vi "2022NewInstrumentationU6_SINGLE_CHANNEL_TEST.vi"() -> ()   [LabVIEW 2021]
panel:
  out "Test 2":dbl(graph)
  in  "Binary 2":bool
  in  "AIN Range":u16(ring) items=["LJ_rgBIP10V", "LJ_rgBIP1V", "LJ_rgBIPP1V", "LJ_rgBIPP01V"]
  in  "FirstFound":bool=TRUE
  in  "Address":string="1"
  out "Error Message 2":string="No Error"
  out "error out":errorcluster
  out "Cold Junction Temp":dbl=41420.0 format="%.6f"
  out "Test":dbl(graph)
  in  "Iterations/Second":i32=1
  in  "Binary":bool
  in  "StreamSettlingFactor":i32
  in  "Resolution Index":u8
  in  "Range Constants":u8[](array[ring])=[0, 0, 0, 0] items=["LJ_rgBIP10V", "LJ_rgBIP1V", "LJ_rgBIPP1V", "LJ_rgBIPP01V"]
  out "Stream Parameters":T1 {"Device Backlog [%]" format="%.2f"}
  in  "PC buffer size (seconds)":dbl=10.0 format="%.2f"
  out "# of iterations":i32
  in  "Scan Rate (Hz)":dbl=1000.0 format="%.3f"
  in  "stop":bool
  out "Error Message":string
  # "This example streams from the first found USB U6."
  # "Data Output For Pressure, Temperature, and Load Sensors"
  # "The + scan list is the positive\nchannels.  For each element in\nthe + list, there must also be\nan element in the - list, which is\nthe negative channels.  For\nsingle-ended channels, put in\n199 for the negative channel.\n\nTo remove an element, right-click\non it, select Data Operations =>\nRemove Element.\n\nTo empty an array, right-click\nnear the edge, select Data\nOperations => Empty Array.\n\nOther useful operations:  From the\nOperate menu are \"Make Current\nValues Default\" and \"Reinitialize\nTo Default\"."
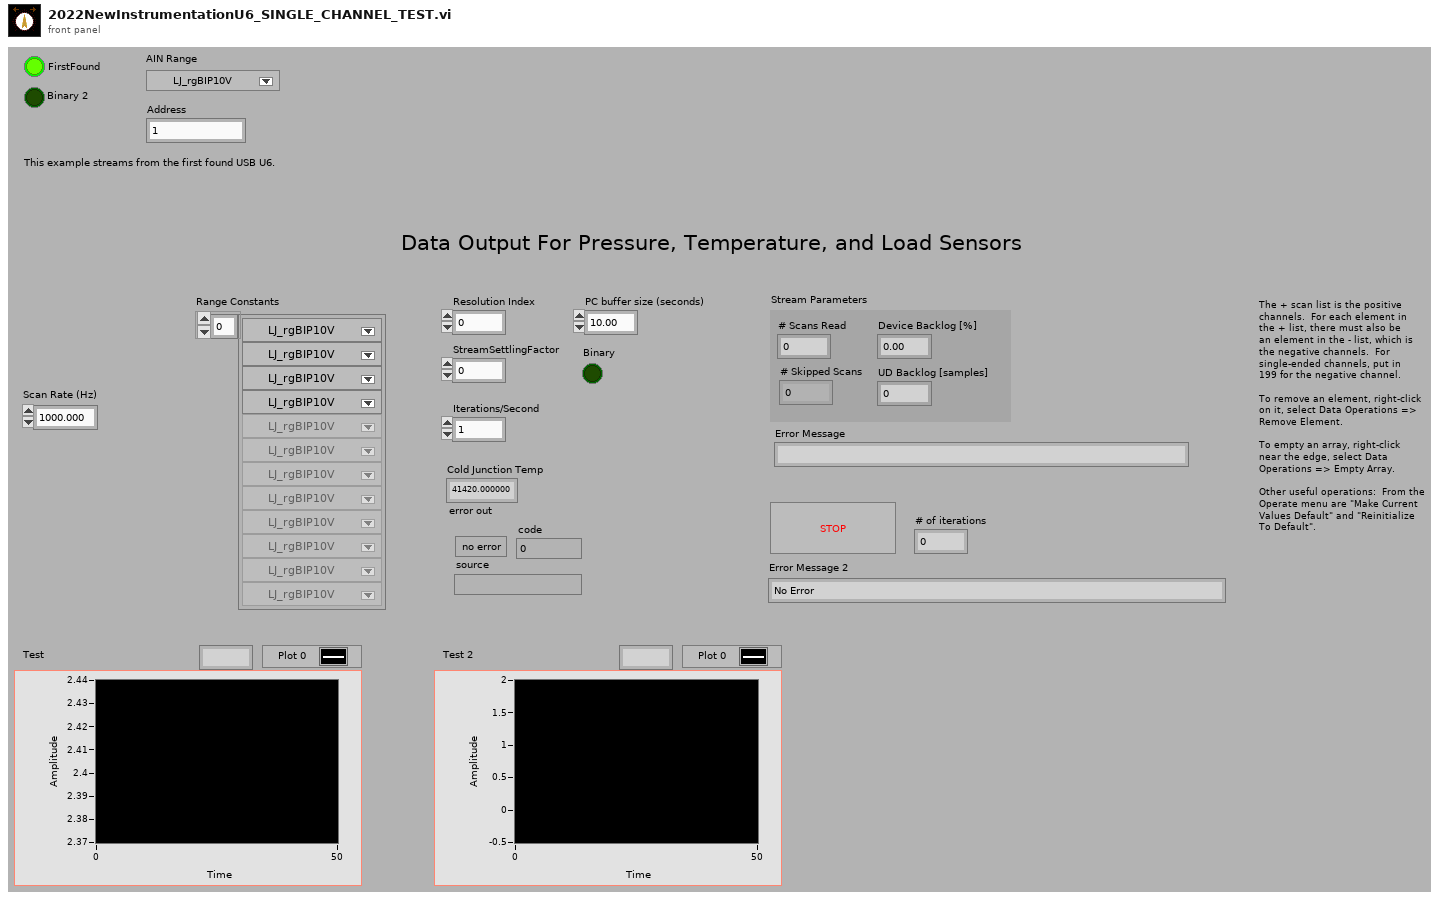
[diagram p1: front panel]
types:
  T1 = cluster{"# Scans Read":i32, "# Skipped Scans":i32, "Device Backlog [%]":dbl, "UD Backlog [samples]":i32}
  T2 = cluster{"PC buffer size (seconds)":dbl, "Resolution Index":u8, "StreamSettlingFactor":i32, "Binary":bool}
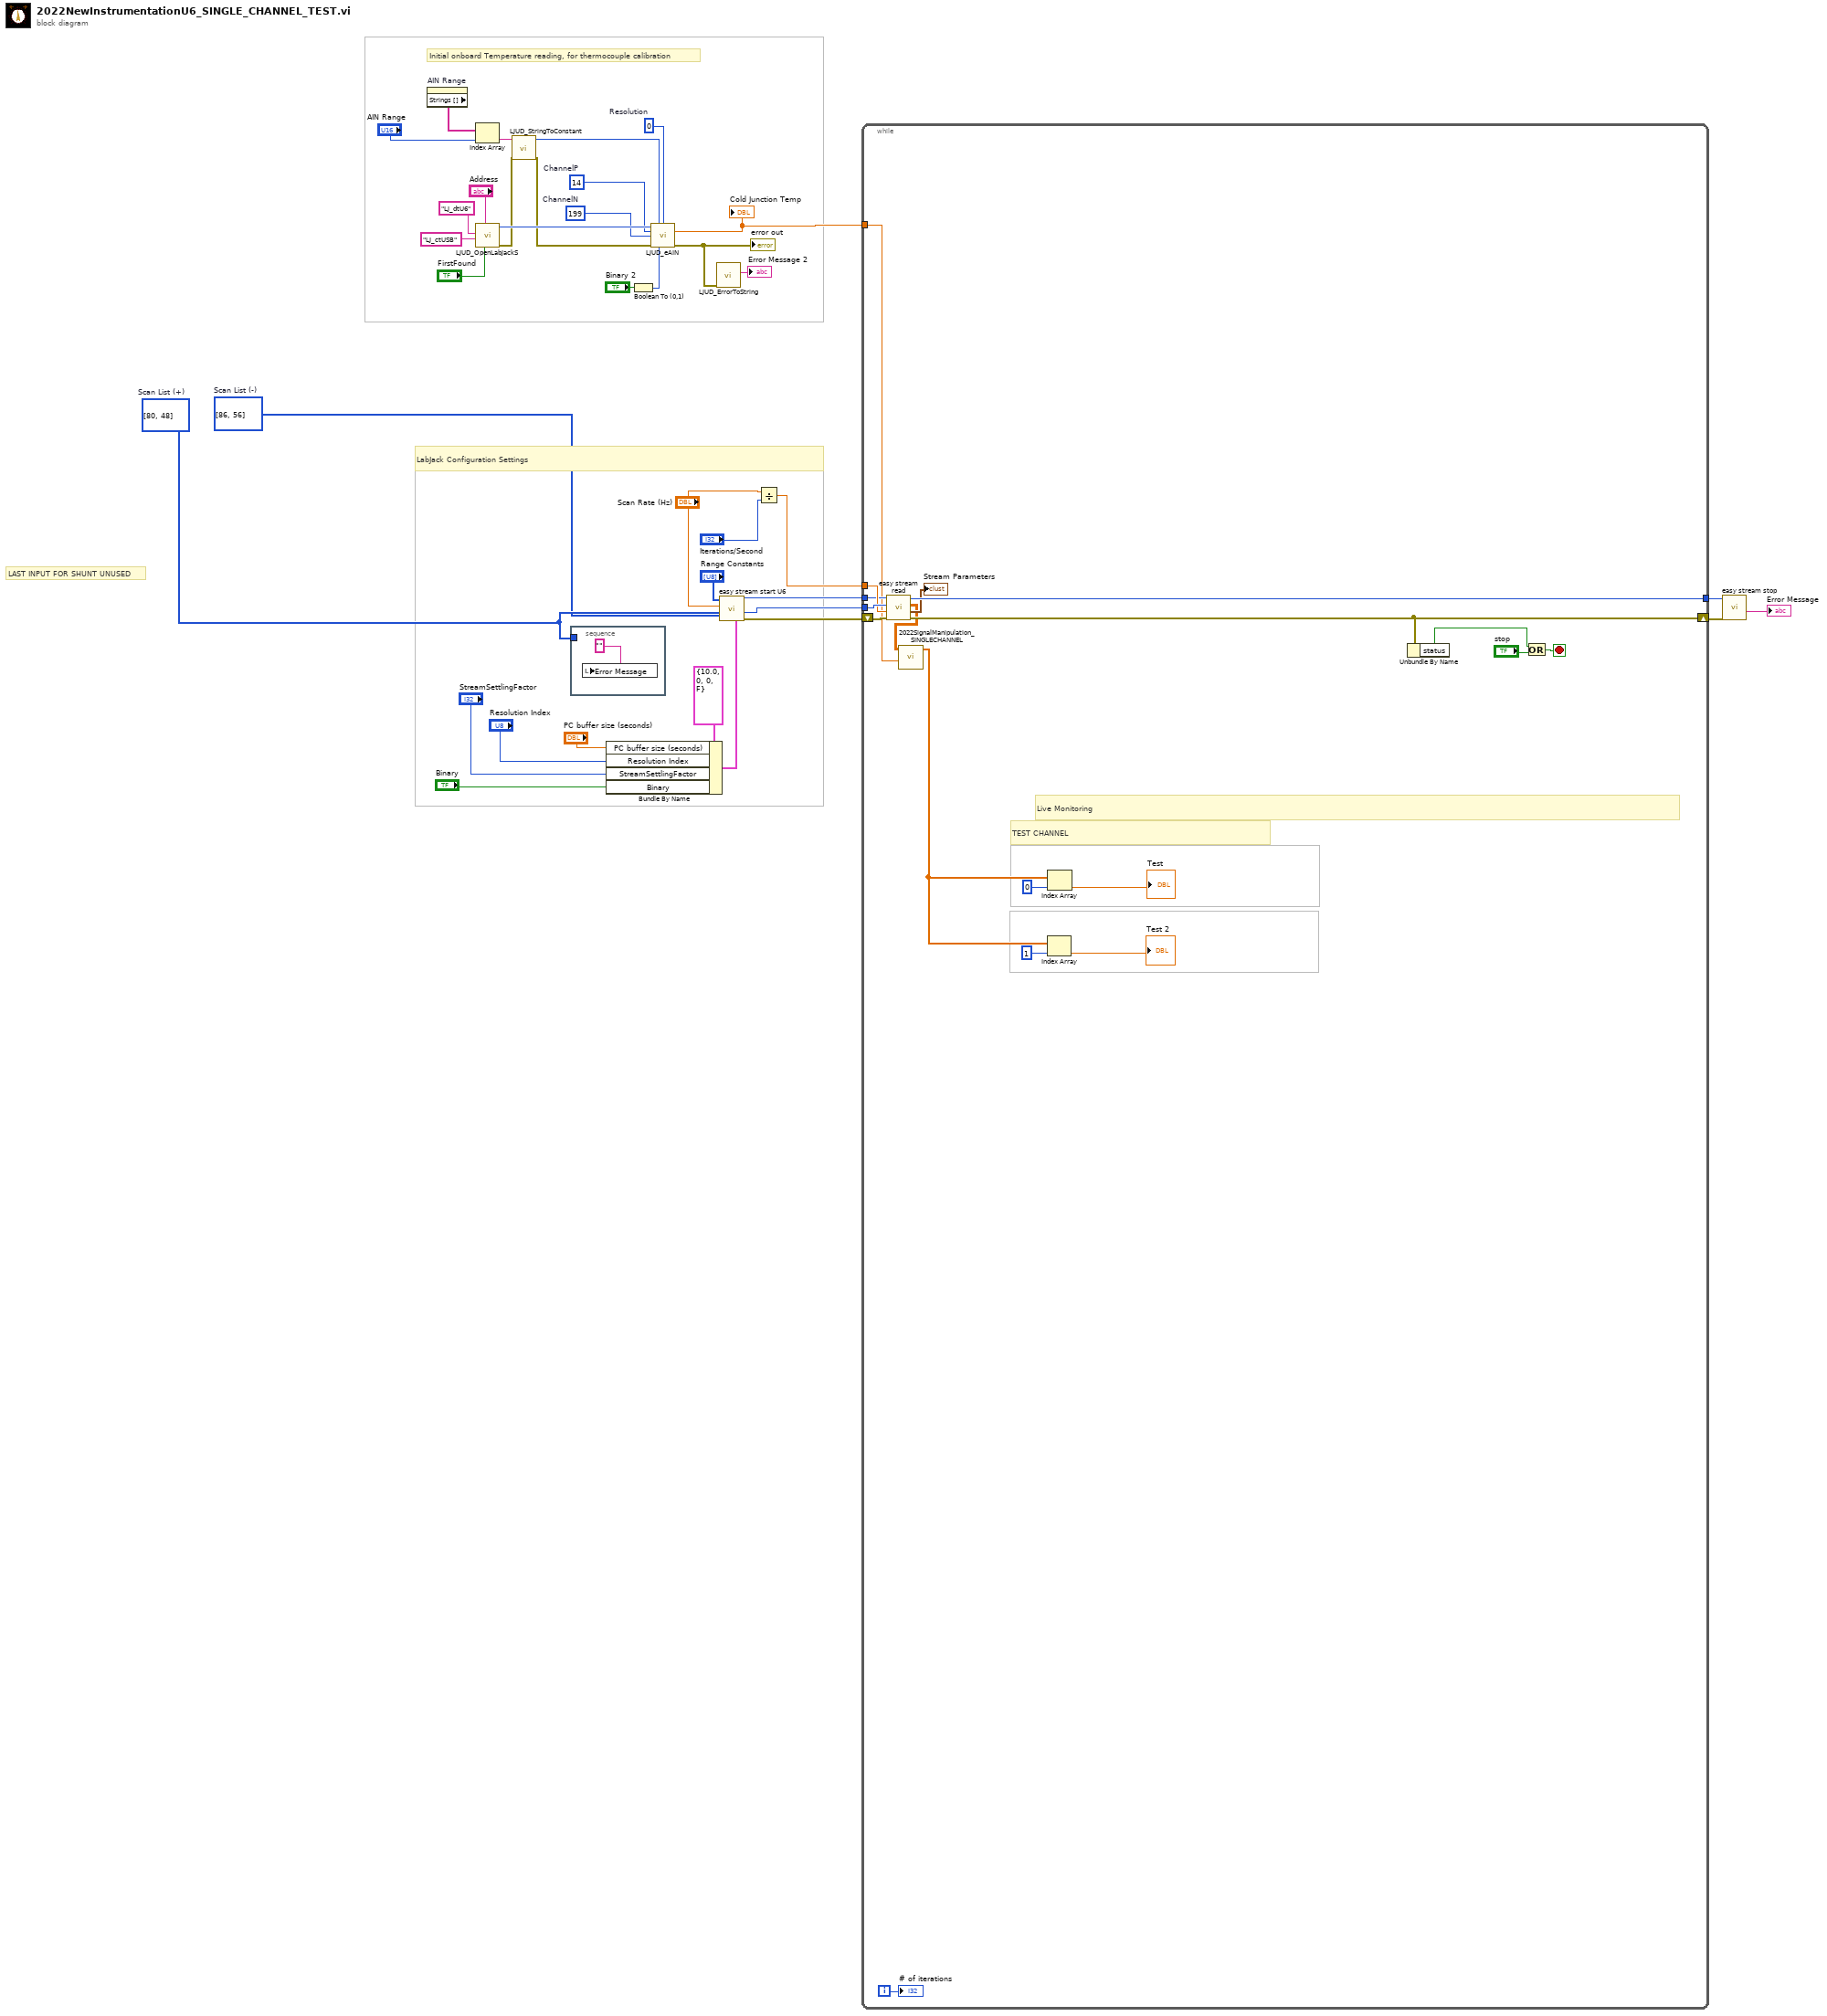
[diagram p0: block diagram]
diagram:
  w12 = 0  # Resolution
  w2 = 199  # ChannelN
  w3 = 14  # ChannelP
  w20 = i32[] [86, 56]  # Scan List (-)
  w21 = i32[] [80, 48]  # Scan List (+)
  # "LAST INPUT FOR SHUNT UNUSED"
  # "LabJack Configuration Settings"
  # "Initial onboard Temperature reading, for thermocouple calibration"
  n1 = property on="AIN Range" class="Ring (strict)"() -> ("Strings []"=w8:string[])  [unwired: 2 in, 2 out]
  n2 = Index Array(array=w8, index="AIN Range") -> (element=w6:string)
  n3 = call "LJUD_OpenLabJackS.vi"("FirstFound"="FirstFound", "Address"="Address", "ConnectionType"="LJ_ctUSB", "DeviceType"="LJ_dtU6") -> ("error out"=w11:errorcluster, "Handle"=w15:i32)  [unwired: 5 in, 1 out]
  n4 = call "LJUD_StringToConstant.vi"("error in"=w11, "String"=w6) -> ("error out"=w10:errorcluster, "Constant Number"=w13:i32)  [unwired: 8 in]
  n5 = stacked-sequence {
    tunnel: w21 -> [_]
    frame #0 {
      n6 = local write "Error Message"("" ("Error Message")) -> ()
    }
  }
  n7 = Bundle By Name(cluster=T2 {"PC buffer size (seconds)"=10.0, "Resolution Index"=0, "StreamSettlingFactor"=0, "Binary"=FALSE} ("Advanced"), "PC buffer size (seconds)"="PC buffer size (seconds)", "Resolution Index"="Resolution Index", "StreamSettlingFactor"="StreamSettlingFactor", "Binary"="Binary") -> (w28:T2)
  n8 = Boolean To (0,1)(Boolean="Binary 2") -> (0, 1=w4:i16)
  n9 = call "LJUD_eAIN.vi"("Handle In"=w15, "Range"=w13, "Resolution"=w12, "ChannelP"=w3, "ChannelN"=w2, "error in"=w10, "Binary"=w4) -> ("Voltage"=w1:dbl, "error out"=w18:errorcluster)  [unwired: 6 in, 1 out]
  "Cold Junction Temp" <- w1
  "error out" <- w18
  n10 = call "LJUD_ErrorToString.vi"("error in"=w18) -> ("String"=→"Error Message 2":string)  [unwired: 10 in]
  n11 = call "easy stream start U6.vi"("Advanced"=w28, "Scan List (-)"=w20, "Scan List (+)"=w21, "Scan Rate (Hz)"="Scan Rate (Hz)", "Range Constants"="Range Constants") -> ("error out"=w37:errorcluster, "# Channels"=w36:i32, "Handle Out"=w35:i32)  [unwired: 3 in, 1 out]
  n12 = Divide(x="Scan Rate (Hz)", y="Iterations/Second") -> (x/y=w32:dbl)
  n13 = while {
    tunnel: w35 -> [w45]
    tunnel: w36 -> [w53]
    shift-left: w37 -> [w54]
    shift-right: [w51] -> w34
    tunnel: w32 -> [w52]
    tunnel: [w50] -> w31
    tunnel: w1 -> [w42]
    i -> [w55]
    stop <- w56 stop-if-true
    # "TEST CHANNEL"
    # "Live Monitoring"
    n14 = call "easy stream read.vi"("error in"=w54, "Scans To Read"=w52, "# Channels In Stream"=w53, "Handle In"=w45) -> ("error out"=w51:errorcluster, "Stream Parameters"=→"Stream Parameters":T1, "Data"=w46:dbl[][], "Handle Out"=w50:i32)  [unwired: 4 in]
    n15 = call "2022SignalManipulation_SINGLECHANNEL.vi"("Cold Junction Temp"=w42, "Data"=w46) -> ("Array"=w39:dbl[])  [unwired: 9 in]
    n16 = Index Array(array=w39, index=1) -> (element=→"Test 2":dbl)
    n17 = Index Array(array=w39, index=0) -> (element=→"Test":dbl)
    n18 = Unbundle By Name(w51) -> ("status"=w48:bool)
    n19 = Or(x=w48, y="stop") -> (x .or. y?=w56:bool)
    "# of iterations" <- w55
  }
  n20 = call "easy stream stop.vi"("error in"=w34, "Handle In"=w31) -> ("Error Message"=→"Error Message":string)  [unwired: 7 in, 2 out]
